vi "CU_addTrainingTrials.vi"(8 "error in (no error)":errorcluster, 10 "Use equal number of trials?":bool, 11 "ClassifierClass in":refnum<class "ClassifierClass.lvclass">) -> (0 "error out":errorcluster, 1 "Num of Trials of each Class":i32[](array[numeric]), 2 "Array of Training Trials out":T1[](array[typedef]), 3 "ClassifierClass out":refnum<class "ClassifierClass.lvclass">)   [LabVIEW 2016, in "Classifier.lvlib" / "ClassifierClass.lvclass"]
uses:
  ClassifierClass.lvclass
  _XML_EEG_Features/XML_FF_Trial.ctl
  ClassifierClass.lvclass/ClassifierClass.ctl
  <vilib>/xml/Close Reference(Node).vi
  _XML_EEG_Features/XML_EEG_Features.lvlib
  <vilib>/xml/NI_XML.lvlib
  Classifier.lvlib
panel:
  # "This VI is a part of BCI Design library, http://www.ru-bci.org \nCopyright © 2020, Sotnikov Peter, All rights reserved. License: GNU GPLv3"
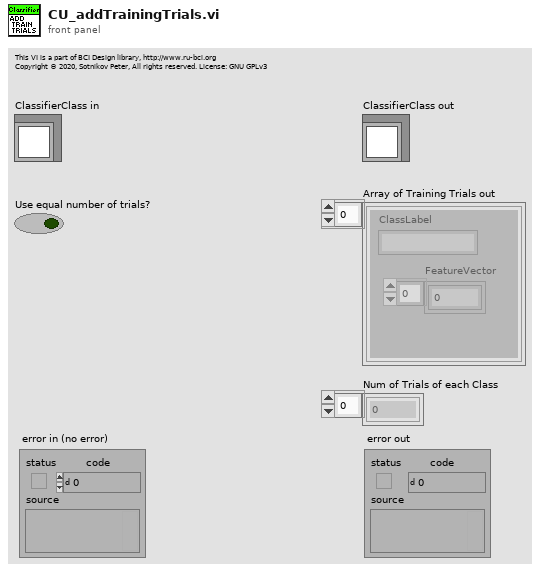
[diagram p1: front panel]
types:
  T1 = typedef "XML_EEG_Features.lvlib/XML_FF_Trial.ctl" = cluster{"ClassLabel":string, "FeatureVector":dbl[]}
  T2 = typedef "XML_EEG_Features.lvlib/XML_FF_Header.ctl" = cluster{"NumberOfTrials":i32, "NumberOfClasses":i32, "FeatureVectorLength":i32, "FeatureExtractionMethod":string}
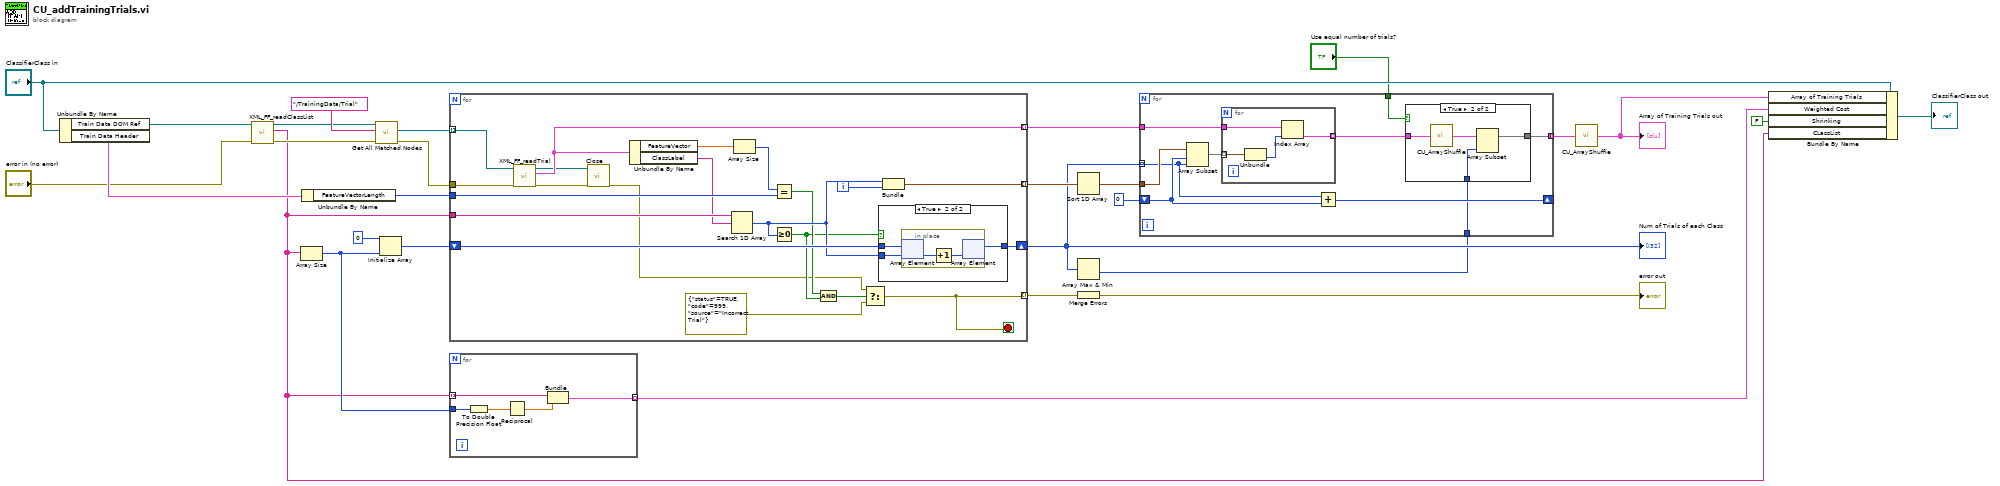
[diagram p0: block diagram]
diagram:
  n1 = Unbundle By Name("ClassifierClass in") -> ("Train Data DOM Ref"=w18:refnum<k20>, "Train Data Header"=w25:T2)
  n2 = call "XML_FF_readClassList.vi"("error in (no error)"="error in (no error)", "DOM document in"=w18) -> ("error out"=w15:errorcluster, "CLassLabels out"=w10:string[], "DOM document out"=w17:refnum<k20>)  [unwired: 7 in]
  n3 = Array Size(array=w10) -> (size(s)=w13:i32)
  n4 = Unbundle By Name(w25) -> ("FeatureVectorLength"=w28:i32)
  n5 = call <vilib>:"Get All Matched Nodes.vi"("error in (no error)"=w15, "XPath expression"="/TrainingData/Trial", "node in"=w17) -> ("error out"=w14:errorcluster, "node result array"=w20:refnum<k20>[])  [unwired: 6 in, 1 out]
  n6 = Initialize Array(0, w13) -> (w11:i32[])
  n7 = for {
    tunnel: w14 -> [w49]
    tunnel: w28 -> [w47]
    tunnel: [w29] -> w27 mode=indexing
    tunnel: [w45] -> w6 mode=indexing
    tunnel: w20 -> [w43] mode=indexing
    shift-right: [w37] -> w8
    shift-left: w11 -> [w38]
    tunnel: w10 -> [w40]
    tunnel: [w35] -> w9 mode=indexing
    i -> [w36]
    stop <- w29 stop-if-true
    n8 = call "XML_FF_readTrial.vi"("error in (no error)"=w49, "DOM document in"=w43) -> ("error out"=w42:errorcluster, "Trial out"=w45:T1, "DOM document out"=w41:refnum<k20>)  [unwired: 7 in]
    n9 = call-poly <vilib>:"Close.vi"("error in (no error)"=w42, "node"=w41) -> ("error out"=w30:errorcluster)  [unwired: 7 in]
    n10 = Unbundle By Name(w45) -> ("FeatureVector"=w46:dbl[], "ClassLabel"=w39:string)
    n11 = Search 1D Array(1D array=w40, element=w39) -> (index of element=w34:i32)  [unwired: 1 in]
    n12 = Array Size(array=w46) -> (size(s)=w48:i32)
    n13 = Equal?(x=w48, y=w47) -> (x = y?=w33:bool)
    n14 = Greater Or Equal To 0?(x=w34) -> (x >= 0?=w32:bool)
    n15 = And(x=w33, y=w32) -> (x .and. y?=w31:bool)
    n16 = Select(t=w30, s=w31, f=errorcluster {"status"=TRUE, "code"=999, "source"="Incorrect Trial"} ("error out")) -> (s? t:f=w29:errorcluster)
    n17 = case shown="True" w32 {
      tunnel: w38 -> [w50 w53]
      tunnel: [w50 w52] -> w37
      tunnel: w34 -> [_ w51]
      frame False {
      }
      frame True {
        n18 = in-place {
          n19 = in-place-array #1(w53, w51) -> (w55:i32)
          n20 = Increment(x=w55) -> (x+1=w54:i32)
          n21 = in-place-array #1(w54) -> (w52:i32[])  [unwired: 1 out]
        }
      }
    }
    n22 = Bundle("index of element"=w34, w36) -> (w35:cluster{"index of element":i32, i32})  [unwired: 1 in]
  }
  "Num of Trials of each Class" <- w8
  n23 = for {
    tunnel: w10 -> [w60] mode=indexing
    tunnel: [w59] -> w22 mode=indexing
    tunnel: w13 -> [w56]
    n24 = To Double Precision Float(number=w56) -> (double precision float=w57:dbl)
    n25 = Reciprocal(x=w57) -> (1/x=w58:dbl)
    n26 = Bundle("node text"=w60, w58) -> (w59:cluster{"node text":string, dbl})  [unwired: 1 in]
  }
  n27 = Sort 1D Array(array=w9) -> (sorted array=w7:cluster{"index of element":i32, i32}[])
  n28 = Array Max & Min(array=w8) -> (min value=w4:i32)  [unwired: 3 out]
  n29 = Merge Errors(w27) -> (→"error out":errorcluster)
  n30 = for {
    tunnel: w8 -> [w65] mode=indexing
    tunnel: w7 -> [w69]
    tunnel: w6 -> [w70]
    shift-right: [w67] -> _
    shift-left: 0 -> [w66]
    tunnel: w4 -> [w63]
    tunnel: [w62] -> w2 mode=concatenating
    tunnel: "Use equal number of trials?" -> [w61]
    n31 = Array Subset(array=w69, index=w66, length=w65) -> (w68:cluster{"index of element":i32, i32}[])
    n32 = for {
      tunnel: w68 -> [w79] mode=indexing
      tunnel: [w77] -> w64 mode=indexing
      tunnel: w70 -> [w76]
      n33 = Unbundle(w79) -> (w78:i32)  [unwired: 1 out]
      n34 = Index Array(array=w76, index=w78) -> (element=w77:T1)
    }
    n35 = Add(x=w65, y=w66) -> (x+y=w67:i32)
    n36 = case shown="True" w61 {
      tunnel: w64 -> [w71 w73]
      tunnel: w63 -> [_ w75]
      tunnel: [w71 w74] -> w62
      frame False {
      }
      frame True {
        n37 = call "CU_ArrayShuffle.vi"("Array in"=w73) -> ("Array out"=w72:T1[])
        n38 = Array Subset(array=w72, length=w75) -> (w74:T1[])  [unwired: 1 in]
      }
    }
  }
  n39 = call "CU_ArrayShuffle.vi"("Array in"=w2) -> ("Array out"=w1:T1[])
  "Array of Training Trials out" <- w1
  n40 = Bundle By Name(cluster="ClassifierClass in", "Array of Training Trials"=w1, "Weighted Cost"=w22, "Shrinking"=FALSE ("Model Options.Shrinking"), "CLassList"=w10) -> (→"ClassifierClass out":refnum<class "ClassifierClass.lvclass">)
